vi "Special Plots Random Generator.vi"(10 "Reuse old data?":bool, 11 "Type of data":T1(ring)) -> (3 "Result":dbl[](array[numeric]) format="%#.6g")   [LabVIEW 2023]
doc: "Generates pseudo-random numbers for the Exploratory Data Analysis.vi example."
uses:
  <vilib>/Analysis/NI_AALBase.lvlib
panel:
  out "Waveform Graph":dbl[](graph)
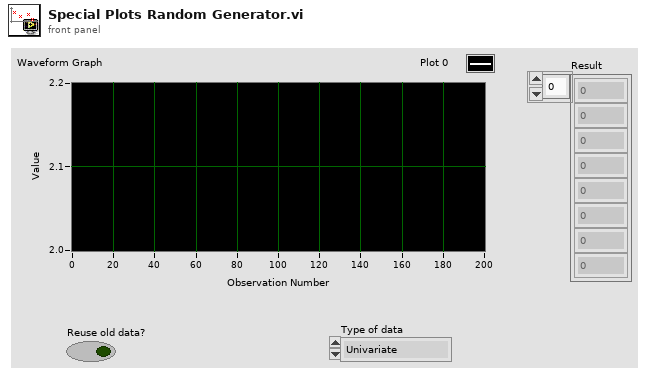
[diagram p1: front panel]
types:
  T1 = enum16{"Univariate", "Linear", "Exponential", "Polynomial", "Sinusoidal", "Constant"}
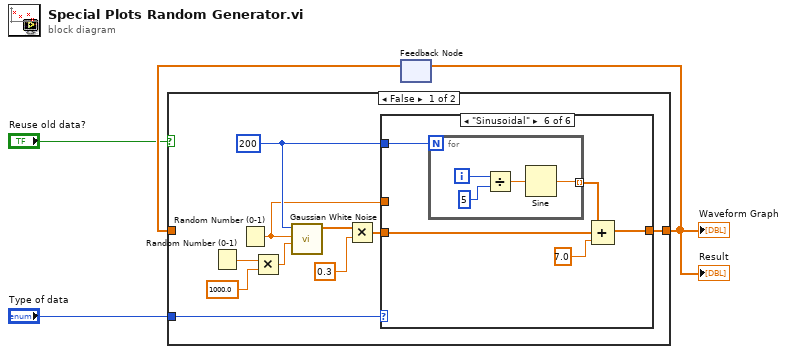
[diagram p0: block diagram]
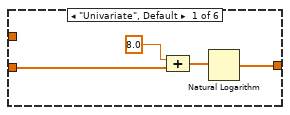
[diagram p2: hidden frame]
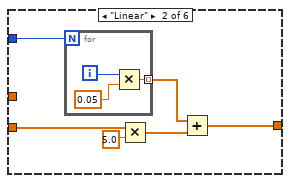
[diagram p3: hidden frame]
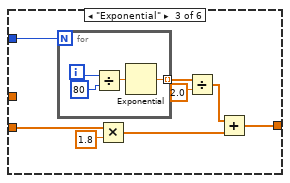
[diagram p4: hidden frame]
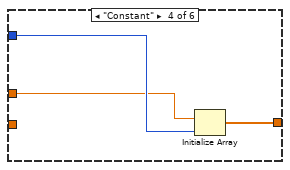
[diagram p5: hidden frame]
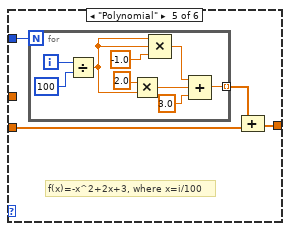
[diagram p6: hidden frame]
diagram:
  n1 = feedback #1() -> (w3:dbl[])  [unwired: 1 in]
  n2 = case shown="False" "Reuse old data?" {
    tunnel: [w9 w65] -> w4
    tunnel: w3 -> [_ w65]
    tunnel: "Type of data" -> [w5 _]
    frame False {
      w11 = 200 ("samples")
      n3 = Random Number (0-1)() -> (number: 0 to 1=w14:dbl)
      n4 = Random Number (0-1)() -> (number: 0 to 1=w8:dbl)
      n5 = Multiply(x=w14, y=1000.0) -> (x*y=w13:dbl)
      n6 = call <vilib>:"Gaussian White Noise.vi"("seed"=w13, "standard deviation"=w8, "samples"=w11) -> ("Gaussian noise pattern"=w12:dbl[])  [unwired: 7 in, 1 out]
      n7 = Multiply(x=w12, y=0.3) -> (x*y=w10:dbl[])
      n8 = case shown="\"Sinusoidal\"" w5 {
        tunnel: w10 -> [w16 w21 w33 _ w44 w60]
        tunnel: [w15 w23 w34 w41 w45 w58] -> w9
        tunnel: w11 -> [_ w24 w35 w42 w46 w57]
        tunnel: w8 -> [_ _ _ w40 _ _]
        frame "Univariate", Default {
          n9 = Compound Arithmetic op=ADD(8.0, w16) -> (w17:dbl[])
          n10 = Natural Logarithm(1:w17) -> (0:w15:dbl[])
        }
        frame "Linear" {
          n11 = for {
            N: w24 -> [_]
            tunnel: [w26] -> w22 mode=indexing
            i -> [w27]
            n12 = Multiply(x=w27, y=0.05) -> (x*y=w26:dbl)
          }
          n13 = Multiply(x=w21, y=5.0) -> (x*y=w20:dbl[])
          n14 = Add(x=w22, y=w20) -> (x+y=w23:dbl[])
        }
        frame "Exponential" {
          n15 = for {
            N: w35 -> [_]
            tunnel: [w37] -> w30 mode=indexing
            i -> [w39]
            n16 = Divide(x=w39, y=80) -> (x/y=w36:dbl)
            n17 = Exponential(1:w36) -> (0:w37:dbl)
          }
          n18 = Multiply(x=w33, y=1.8) -> (x*y=w32:dbl[])
          n19 = Divide(x=w30, y=2.0) -> (x/y=w29:dbl[])
          n20 = Add(x=w29, y=w32) -> (x+y=w34:dbl[])
        }
        frame "Constant" {
          n21 = Initialize Array(w40, w42) -> (w41:dbl[])
        }
        frame "Polynomial" {
          # "f(x)=-x^2+2x+3, where x=i/100"
          n22 = for {
            N: w46 -> [_]
            tunnel: [w51] -> w43 mode=indexing
            i -> [w49]
            n23 = Divide(x=w49, y=100) -> (x/y=w50:dbl)
            n24 = Multiply(x=2.0, y=w50) -> (x*y=w55:dbl)
            n25 = Compound Arithmetic op=MULTIPLY(w50, w50, -1.0 ("value")) -> (w53:dbl)
            n26 = Compound Arithmetic op=ADD(w53, w55, 3.0) -> (w51:dbl)
          }
          n27 = Compound Arithmetic op=ADD(w43, w44) -> (w45:dbl[])
        }
        frame "Sinusoidal" {
          n28 = for {
            N: w57 -> [_]
            tunnel: [w61] -> w59 mode=indexing
            i -> [w64]
            n29 = Divide(x=w64, y=5) -> (x/y=w62:dbl)
            n30 = Sine(x=w62) -> (sin(x)=w61:dbl)
          }
          n31 = Compound Arithmetic op=ADD(w59, w60, 7.0) -> (w58:dbl[])
        }
      }
    }
    frame True {
      # "Reused old data or this is the first time the VI is run"
    }
  }
  "Result" <- w4
  "Waveform Graph" <- w4
  n32 = feedback-in #1(w4) -> ()
